vi "Generate Holonomic Thetas.vi"(6 "WayPoints":T1, 8 "time unflat":cluster{dbl[]}[](array[cluster]), 9 "dt":dbl, 11 "Angular Limits":T2={"Velocity (deg/s)"=6.0, "Accel (deg/s^2)"=15.0, "Jerk (deg/s^3)"=150.0} {"Jerk (deg/s^3)" min=0.0 step=1.0; "Accel (deg/s^2)" min=0.0; "Velocity (deg/s)" min=0.0}) -> (2 "X":dbl[](array[numeric]), 3 "V":dbl[](array[numeric]))   [LabVIEW 2025]
uses:
  Types/Angluar Limits.ctl
  Types/Waypoints.ctl
panel:
  out "x*y 2":dbl
  out "x*y":dbl
  out "Waveform Chart 2":dbl[](graph)
  out "Waveform Chart":dbl[](graph)
  out "output variable":i32
  out "size(s) 2":i32
  out "size(s)":i32
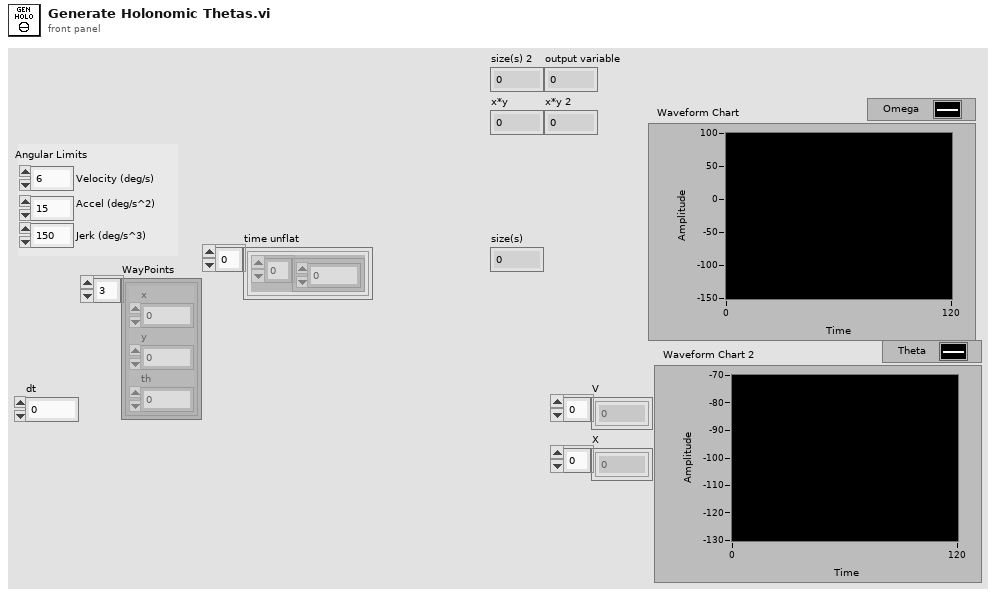
[diagram p1: front panel]
types:
  T1 = typedef "Waypoints.ctl" = cluster{"x":sgl, "y":sgl, "th":sgl}[]
  T2 = typedef "Angluar Limits.ctl" = cluster{"Velocity (deg/s)":dbl, "Accel (deg/s^2)":dbl, "Jerk (deg/s^3)":dbl}
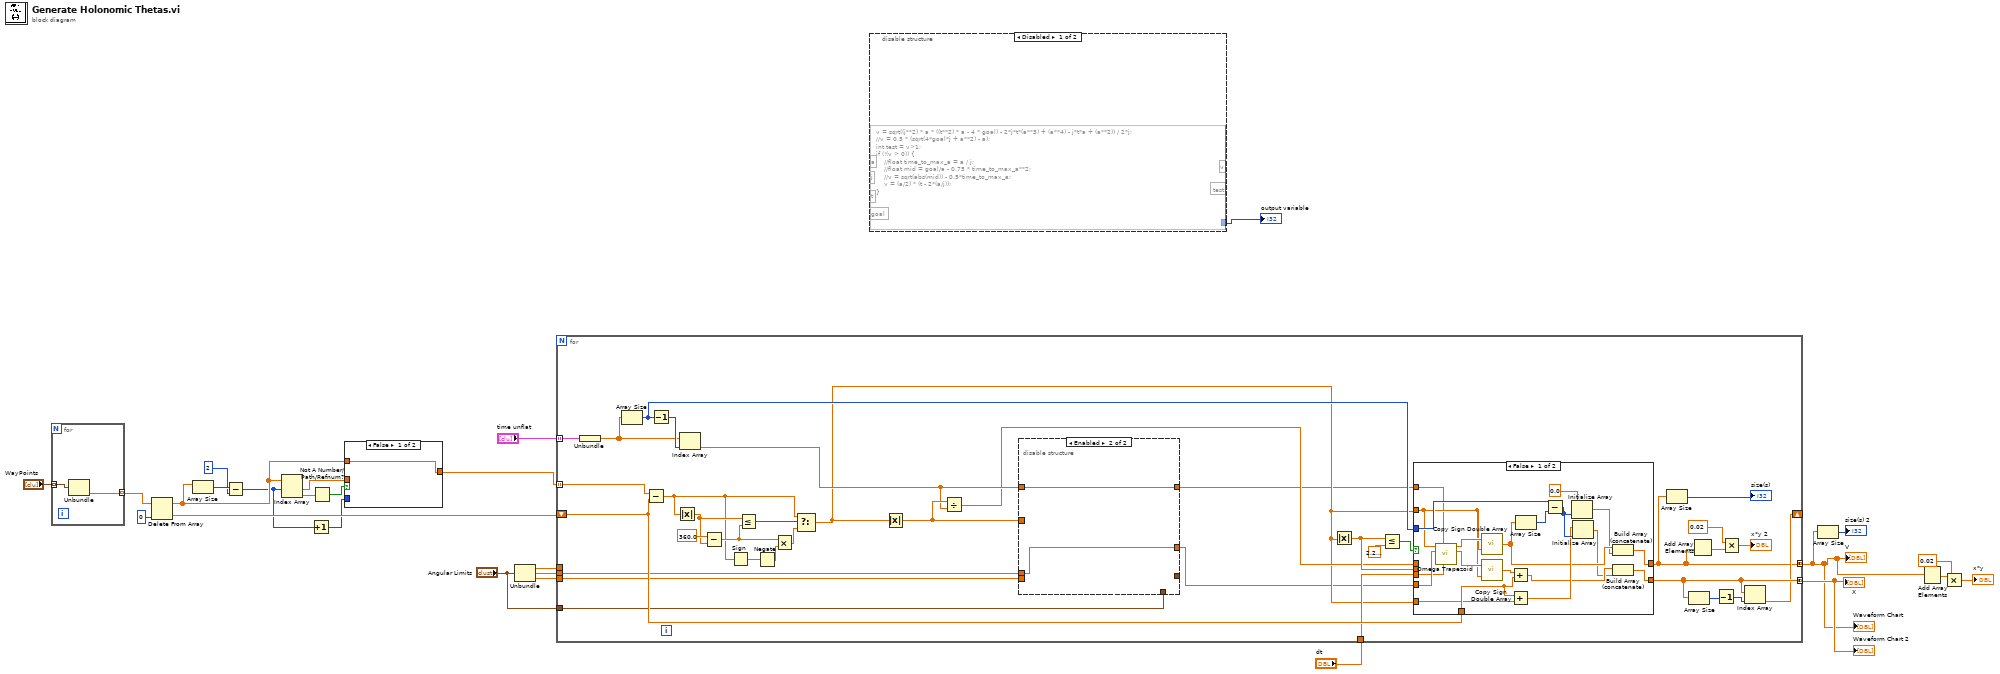
[diagram p0: block diagram]
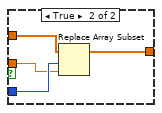
[diagram p2: hidden frame]
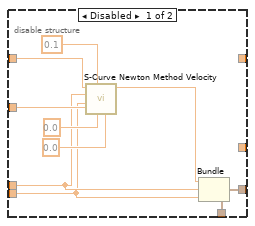
[diagram p4: hidden frame]
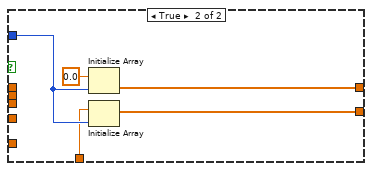
[diagram p5: hidden frame]
diagram:
  n1 = for {
    tunnel: "WayPoints" -> [w28] mode=indexing
    tunnel: [w27] -> w18 mode=indexing
    n2 = Unbundle(w28) -> ("th"=w27:sgl)  [unwired: 2 out]
  }
  n3 = Delete From Array(array=w18, index=0) -> (deleted portion=w16:sgl, array with subset deleted=w14:sgl[])  [unwired: 1 in]
  n4 = Array Size(array=w14) -> (size(s)=w13:i32)
  n5 = Subtract(x=w13, y=2) -> (x-y=w10:i32)
  n6 = Index Array(array=w14, index #1=w10) -> (element #1=w8:sgl, element #2=w11:sgl)  [unwired: 1 in]
  n7 = Increment(x=w10) -> (x+1=w9:i32)
  n8 = Not A Number/Path/Refnum?(number/path/refnum=w11) -> (NaN/Path/Refnum?=w15:bool)
  n9 = case shown="False" w15 {
    tunnel: w14 -> [w29 w33]
    tunnel: w9 -> [_ w32]
    tunnel: w8 -> [_ w31]
    tunnel: [w29 w30] -> w7
    frame False {
    }
    frame True {
      n10 = Replace Array Subset(array=w33, new element=w31, index=w32) -> (w30:sgl[])
    }
  }
  n11 = Unbundle("Angular Limits") -> ("Velocity (deg/s)"=w26:dbl, "Accel (deg/s^2)"=w24:dbl, "Jerk (deg/s^3)"=w25:dbl)
  n12 = for {
    tunnel: w26 -> [_]
    tunnel: w25 -> [w54]
    tunnel: w24 -> [w55]
    tunnel: w7 -> [w65] mode=indexing
    shift-right: [w57] -> _
    shift-left: w16 -> [w61]
    tunnel: "dt" -> [w52]
    tunnel: "time unflat" -> [w64] mode=indexing
    tunnel: [w37] -> w4 mode=concatenating
    tunnel: [w60] -> w5 mode=concatenating
    tunnel: "Angular Limits" -> [w56]
    n13 = Unbundle(w64) -> (w63:dbl[])
    n14 = Array Size(array=w63) -> (size(s)=w66:i32)
    n15 = Subtract(x=w65, y=w61) -> (x-y=w44:dbl)
    n16 = Decrement(x=w66) -> (x-1=w67:i32)
    n17 = Absolute Value(x=w44) -> (abs(x)=w46:dbl)
    n18 = Index Array(array=w63, index=w67) -> (element=w50:dbl)
    n19 = Subtract(x=360.0, y=w46) -> (x-y=w45:dbl)
    n20 = Sign(1:w44) -> (0:w43:dbl)
    n21 = Less Or Equal?(x=w46, y=w45) -> (x <= y?=w47:bool)
    n22 = Negate(x=w43) -> (-x=w42:dbl)
    n23 = Multiply(x=w45, y=w42) -> (x*y=w41:dbl)
    n24 = Select(t=w44, s=w47, f=w41) -> (s? t:f=w40:dbl)
    n25 = Absolute Value(x=w40) -> (abs(x)=w51:dbl)
    n26 = Divide(x=w51, y=w50) -> (x/y=w49:dbl)
    n27 = disable-structure shown="Enabled" {
      disable-tunnel: w50 -> [w79 w80]
      disable-tunnel: w51 -> [w75 _]
      disable-tunnel: w56 -> [w73 _]
      disable-tunnel: w55 -> [w72 w81]
      disable-tunnel: w54 -> [w71 _]
      disable-tunnel: [w70 _] -> _
      disable-tunnel: [_ w81] -> w39
      disable-tunnel: [_ w80] -> w38
      frame Disabled {
        n28 = call "S-Curve Newton Method Velocity.vi"("v_f"=0.0, "v_i"=0.0, "err"=0.1, "g"=w75, "j"=w71, "a"=w72, "t"=w79) -> ("v_out"=w74:dbl)  [unwired: 4 in]
        n29 = Bundle(cluster=w73, "Velocity (deg/s)"=w74, "Accel (deg/s^2)"=w72, "Jerk (deg/s^3)"=w71) -> (w70:T2)
      }
      frame Enabled {
      }
    }
    n30 = Absolute Value(x=w40) -> (abs(x)=w53:dbl)
    n31 = Less Or Equal?(x=w53, y=2.220446049250313e-16) -> (x <= y?=w68:bool)
    n32 = case shown="False" w68 {
      tunnel: [w92 w106] -> w37
      tunnel: [w89 w104] -> w60
      tunnel: w66 -> [w100 w103]
      tunnel: w61 -> [w96 w102]
      tunnel: w40 -> [w83 _]
      tunnel: w40 -> [w88 _]
      tunnel: w53 -> [_ _]
      tunnel: w52 -> [w84 _]
      tunnel: w49 -> [_ _]
      tunnel: w39 -> [w85 _]
      tunnel: w38 -> [w82 _]
      frame False {
        n33 = call "Omega Trapezoid.vi"("dt"=w84, "ttot"=w82, "a"=w85, "g"=w83) -> ("Thetas"=w86:dbl[], "Omegas"=w87:dbl[])  [unwired: 6 in]
        n34 = call "Copy Sign Double Array.vi"("y"=w83, "x"=w86) -> ("x out"=w101:dbl[])
        n35 = call "Copy Sign Double Array.vi"("y"=w83, "x"=w87) -> ("x out"=w94:dbl[])
        n36 = Add(x=w101, y=w96) -> (x+y=w91:dbl[])
        n37 = Add(x=w96, y=w88) -> (x+y=w95:dbl)
        n38 = Array Size(array=w94) -> (size(s)=w99:i32)
        n39 = Subtract(x=w100, y=w99) -> (x-y=w98:i32)
        n40 = Initialize Array(0.0 ("element"), w98) -> (w93:dbl[])
        n41 = Initialize Array(w95, w98) -> (w90:dbl[])
        n42 = Build Array (concatenate)(w94, w93) -> (w92:dbl[])
        n43 = Build Array (concatenate)(w91, w90) -> (w89:dbl[])
      }
      frame True {
        n44 = Initialize Array(0.0 ("element"), w103) -> (w106:dbl[])
        n45 = Initialize Array(w102, w103) -> (w104:dbl[])
      }
    }
    n46 = Array Size(array=w37) -> (size(s)=→"size(s)":i32)
    n47 = Array Size(array=w60) -> (size(s)=w59:i32)
    n48 = Add Array Elements(numeric array=w37) -> (sum=w36:dbl)
    n49 = Decrement(x=w59) -> (x-1=w58:i32)
    n50 = Multiply(x=0.02 ("y"), y=w36) -> (x*y=→"x*y 2":dbl)
    n51 = Index Array(array=w60, index=w58) -> (element=w57:dbl)
  }
  "V" <- w4
  "X" <- w5
  "Waveform Chart" <- w4
  "Waveform Chart 2" <- w5
  n52 = disable-structure shown="Disabled" {
    disable-tunnel: [w107 _] -> w19
    frame Disabled {
      n53 = formula code="v = sqrt((j**2) * a * ((t**2) * a - 4 * goal) - 2*j*t*(a**3) + (a**4) - j*t*a + (a**2)) / 2*j;\n//v = 0.5 * (sqrt(4*goal*j + a**2) - a);\nint test = v>1;\nif (!(v > 0)) {\n    //float time_to_max_a = a / j;\n    //float mid = goal/a - 0.75 * time_to_max_a**2;\n    //v = sqrt(abs(mid)) - 0.5*time_to_max_a;\n    v = (a/2) * (t - 2*(a/j));\n}"() -> ("test"=w107:i32)  [unwired: 4 in, 1 out]
    }
    frame Enabled {
    }
  }
  "output variable" <- w19
  n54 = Array Size(array=w4) -> (size(s)=→"size(s) 2":i32)
  n55 = Add Array Elements(numeric array=w4) -> (sum=w3:dbl)
  n56 = Multiply(x=w3, y=0.02) -> (x*y=→"x*y":dbl)
